vi "Bordeaux to Botpose Convert Coordinates.vi"(11 "Pos In":cluster{"x":dbl, "y":dbl}) -> (3 "Pos Out":cluster{dbl[unit], dbl[unit]})   [LabVIEW 2025]
uses:
  <vilib>/Rock Robotics/WPI/DriverStation/WPI_DriverStationAllianceInfo.ctl
panel:
  out "new y":dbl[unit]
  out "new x":dbl[unit]
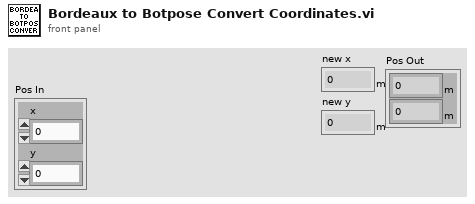
[diagram p1: front panel]
types:
  T1 = typedef "WPI_DriverStationAllianceInfo.ctl" = enum16{"Red", "Blue", "Invalid"}
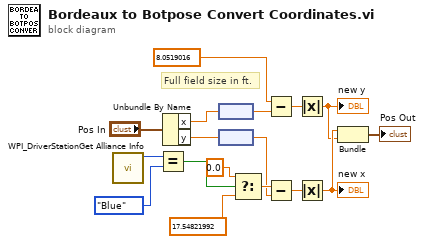
[diagram p0: block diagram]
diagram:
  # "Full field size in ft."
  n1 = call <vilib>:"WPI_DriverStationGet Alliance Info.vi"() -> ("Alliance"=w2:T1)  [unwired: 6 in, 5 out]
  n2 = Equal?(x=w2, y=WPI_DriverStationAllianceInfo."Blue") -> (x = y?=w14:bool)
  n3 = Unbundle By Name("Pos In") -> ("x"=w16:dbl, "y"=w17:dbl)
  n4 = node(w16) -> (w6:dbl[unit])
  n5 = node(w17) -> (w12:dbl[unit])
  n6 = Select(t=dbl[unit] 0.0, s=w14, f=dbl[unit] 17.54821992) -> (s? t:f=w13:dbl[unit])
  n7 = Subtract(x=dbl[unit] 8.0519016, y=w6) -> (x-y=w8:dbl[unit])
  n8 = Subtract(x=w13, y=w12) -> (x-y=w9:dbl[unit])
  n9 = Absolute Value(x=w8) -> (abs(x)=w4:dbl[unit])
  "new y" <- w4
  n10 = Absolute Value(x=w9) -> (abs(x)=w7:dbl[unit])
  "new x" <- w7
  n11 = Bundle(w7, w4) -> (→"Pos Out":cluster{dbl[unit], dbl[unit]})  [unwired: 1 in]
